vi "Load Config.vi"(6 "Constants":refnum<class "Sequence Constants.lvclass">, 8 "error in (no error)":refnum<class "MultiErrors.lvclass">, 10 "Config Element":refnum<class "Config Element.lvclass">, 11 "LowLimit Condition Config in":refnum<class "LowLimit Condition Config.lvclass">) -> (0 "error out":refnum<class "MultiErrors.lvclass">, 3 "LowLimit Condition Config out":refnum<class "LowLimit Condition Config.lvclass">)   [LabVIEW 2020, in "VolatusSeqConfig.lvlib" / "LowLimit Condition Config.lvclass"]
uses:
  LowLimit Condition Config.lvclass
  VolatusErrorUtilities/MultiErrors/MultiErrors.lvclass
  lv-cdm/CDM-Config/Config Element/Config Element.lvclass
  Sequence Constants/Sequence Constants.lvclass
  LowLimit Condition Config.lvclass/LowLimit Condition Config.ctl
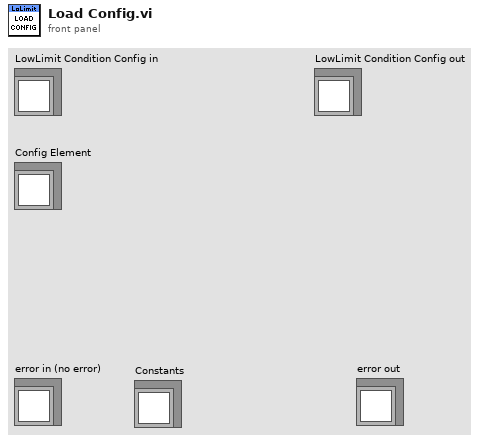
[diagram p1: front panel]
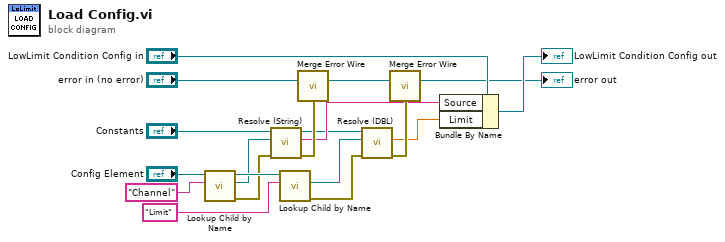
[diagram p0: block diagram]
diagram:
  n1 = call "Lookup Child by Name.vi"("Name"="Channel", "Config Element in"="Config Element") -> ("error out"=w6:errorcluster, "Child"=w12:refnum<class "Config Element.lvclass">, "Config Element out"=w14:refnum<class "Config Element.lvclass">)  [unwired: 6 in, 1 out]
  n2 = call "Resolve (String).vi"("error in (no error)"=w6, "Element"=w12, "Sequence Constants in"="Constants") -> ("error out"=w18:errorcluster, "String Value"=w8:string, "Sequence Constants out"=w2:refnum<class "Sequence Constants.lvclass">)  [unwired: 6 in]
  n3 = call "Lookup Child by Name.vi"("Name"="Limit", "Config Element in"=w14) -> ("error out"=w5:errorcluster, "Child"=w11:refnum<class "Config Element.lvclass">)  [unwired: 6 in, 2 out]
  n4 = call "Merge Error Wire.vi"("error in (no error)"=w18, "MultiErrors in"="error in (no error)") -> ("MultiErrors out"=w4:refnum<class "MultiErrors.lvclass">)  [unwired: 13 in]
  n5 = call "Resolve (DBL).vi"("error in (no error)"=w5, "Element"=w11, "Sequence Constants in"=w2) -> ("error out"=w19:errorcluster, "DBL Value"=w7:dbl)  [unwired: 6 in, 1 out]
  n6 = call "Merge Error Wire.vi"("error in (no error)"=w19, "MultiErrors in"=w4) -> ("MultiErrors out"=→"error out":refnum<class "MultiErrors.lvclass">)  [unwired: 13 in]
  n7 = Bundle By Name(cluster="LowLimit Condition Config in", "Source"=w8, "Limit"=w7) -> (→"LowLimit Condition Config out":refnum<class "LowLimit Condition Config.lvclass">)
